vi "Read Thermocouple Temps.vi"(10 "Accuracy Selector":enum16{"High Accuracy", "High Speed"}(ring)) -> (0 "data":dynamicdata(waveform), 2 "Values":dbl[][](array[numeric]), 3 "Names":string[](array[string]))   [LabVIEW 2021]
uses:
  <vilib>/express/express shared/transition.llb/Dynamic To Waveform Array.vi
  <vilib>/express/express signal manip/GetorSetDDTAttributes/Get DDT Attributes/Get DDT Properties.xnode
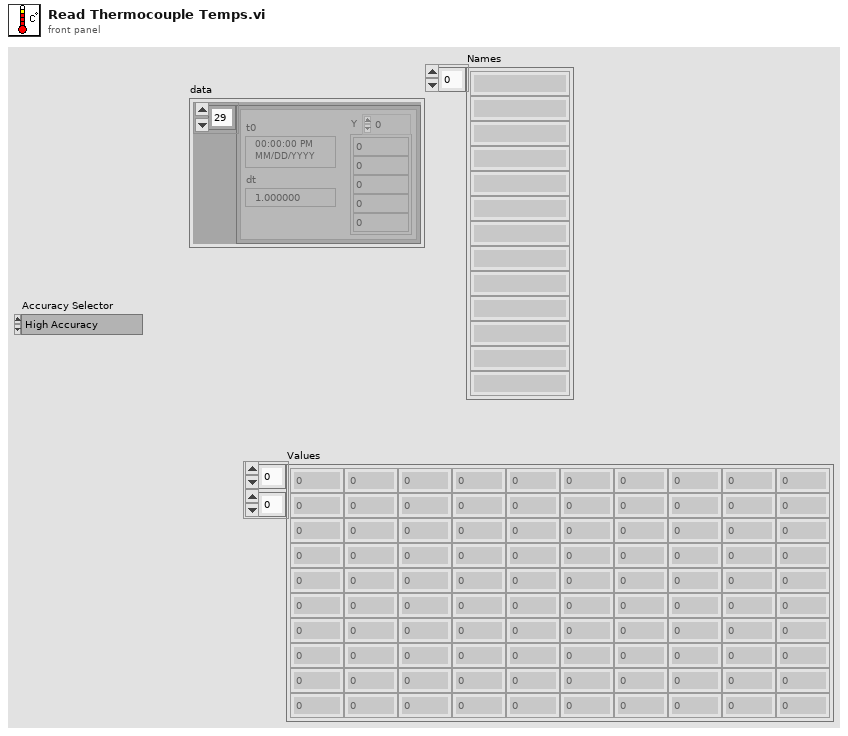
[diagram p1: front panel]
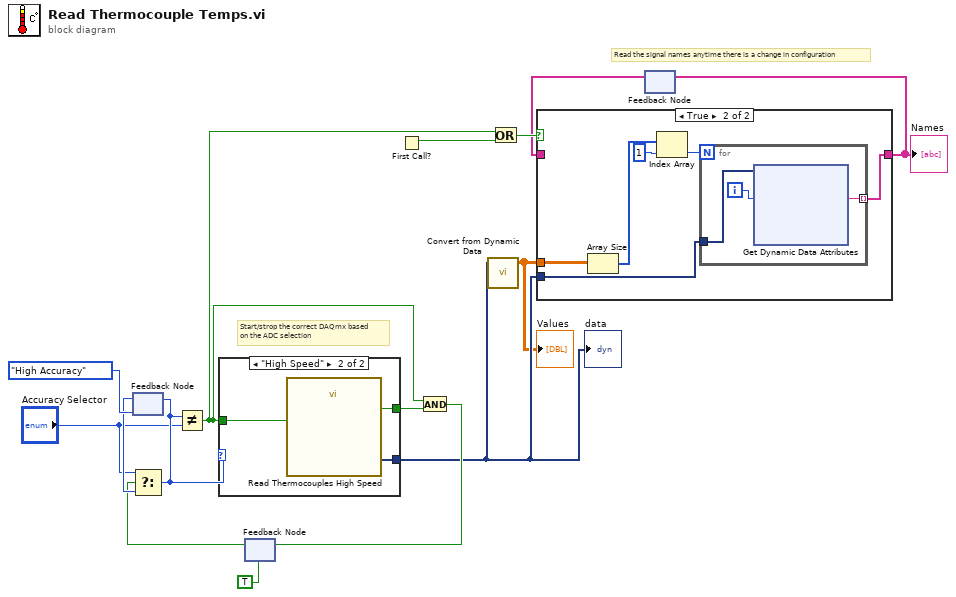
[diagram p0: block diagram]
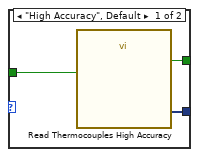
[diagram p3: hidden frame]
diagram:
  # "Start/strop the correct DAQmx based \non the ADC selection"
  # "Read the signal names anytime there is a change in configuration"
  n1 = feedback #1(enum16{"High Accuracy", "High Speed"}."High Accuracy" ("Thermocouple selector")) -> (w14:enum16{"High Accuracy", "High Speed"})
  n2 = feedback #2(TRUE) -> (w10:bool)
  n3 = Select(t="Accuracy Selector", s=w10, f=w14) -> (s? t:f=w12:enum16{"High Accuracy", "High Speed"})
  n4 = feedback-in #1(w12) -> ()
  n5 = Not Equal?(x=w12, y="Accuracy Selector") -> (x != y?=w6:bool)
  n6 = case shown="\"High Speed\"" w12 {
    tunnel: [w18 w21] -> w13
    tunnel: [w17 w20] -> w4
    tunnel: w6 -> [w16 w19]
    frame "High Accuracy", Default {
      n7 = call "Read Thermocouples High Accuracy"("stop (F)"=w16) -> ("data"=w17:dynamicdata, "stopped"=w18:bool)  [unwired: 15 in, 2 out]
    }
    frame "High Speed" {
      n8 = call "Read Thermocouples High Speed"("stop (F)"=w19) -> ("data"=w20:dynamicdata, "stopped"=w21:bool)  [unwired: 15 in, 2 out]
    }
  }
  "data" <- w4
  n9 = First Call?() -> (First Call?: T/F=w7:bool)
  n10 = And(x=w6, y=w13) -> (x .and. y?=w11:bool)
  n11 = feedback-in #2(w11) -> ()
  n12 = call "Convert from Dynamic Data"("Dynamic Data Type"=w4) -> ("Array"=w1:dbl[][])  [unwired: 3 in]
  "Values" <- w1
  n13 = Or(x=w6, y=w7) -> (x .or. y?=w5:bool)
  n14 = feedback #3() -> (w2:string[])  [unwired: 1 in]
  n15 = case shown="True" w5 {
    tunnel: w4 -> [_ w28]
    tunnel: w1 -> [_ w27]
    tunnel: [w22 w23] -> w3
    tunnel: w2 -> [w22 _]
    frame False {
    }
    frame True {
      n16 = Array Size(array=w27) -> (size(s)=w26:i32[])
      n17 = Index Array(array=w26, index=1) -> (element=w24:i32)
      n18 = for {
        N: w24 -> [_]
        tunnel: w28 -> [w31]
        tunnel: [w30] -> w23 mode=indexing
        i -> [w29]
        n19 = xnode "Get Dynamic Data Attributes"("Signals In"=w31, "Signal Index"=w29) -> ("Signal Name"=w30:string)  [unwired: 1 in, 2 out]
      }
    }
  }
  "Names" <- w3
  n20 = feedback-in #3(w3) -> ()
